vi "Day 01 (Part One).vi"() -> ()   [LabVIEW 2021]
panel:
  out "result":i32
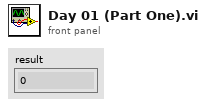
[diagram p1: front panel]
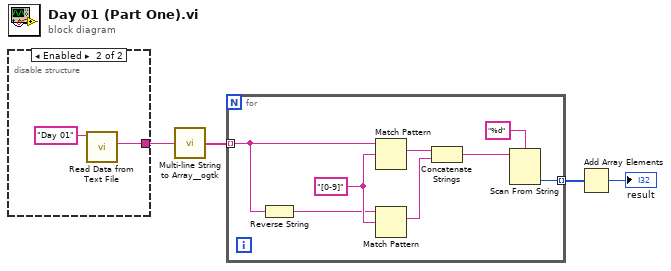
[diagram p0: block diagram]
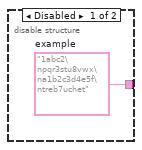
[diagram p2: hidden frame]
diagram:
  n1 = disable-structure shown="Enabled" {
    disable-tunnel: [w5 w6] -> w1
    frame Disabled {
      w5 = "1abc2\npqr3stu8vwx\na1b2c3d4e5f\ntreb7uchet"  # example
    }
    frame Enabled {
      n2 = call "Read Data from Text File.vi"("Subfolder"="Day 01") -> ("data"=w6:string)  [unwired: 10 in]
    }
  }
  n3 = call <userlib>:"Multi-line String to Array__ogtk.vi"("string"=w1) -> ("lines"=w4:string[])
  n4 = for {
    tunnel: w4 -> [w13] mode=indexing
    tunnel: [w8] -> w3 mode=indexing
    w15 = "[0-9]" ("regular expression")
    n5 = Reverse String(1:w13) -> (0:w14:string)
    n6 = Match Pattern(string=w13, regular expression=w15) -> (match substring=w12:string)  [unwired: 1 in, 3 out]
    n7 = Match Pattern(string=w14, regular expression=w15) -> (match substring=w11:string)  [unwired: 1 in, 3 out]
    n8 = Concatenate Strings(w12, w11) -> (w9:string)
    n9 = Scan From String(format string="%d", input string=w9) -> (output 1=w8:i32)  [unwired: 3 in, 3 out]
  }
  n10 = Add Array Elements(numeric array=w3) -> (sum=→"result":i32)
